vi "Write Attribute.vi"(4 "Private?":bool, 5 "Update Pointer?":bool, 6 "Pointer?":bool, 7 "Linked List ID":string, 8 "error in (no error)":errorcluster, 9 "Attribute":variant, 10 "Attribute Name":string, 11 "Linked List in":refnum<class "Linked List.lvclass">) -> (0 "error out":errorcluster, 1 "Replaced?":bool, 2 "Unique ID":string, 3 "Linked List out":refnum<class "Linked List.lvclass">)   [LabVIEW 2019, in "Linked Lists.lvlib" / "Linked List.lvclass"]
uses:
  <vilib>/gpm_packages/@cs/linked-list/Source/Linked List/Linked List/Linked List.lvclass
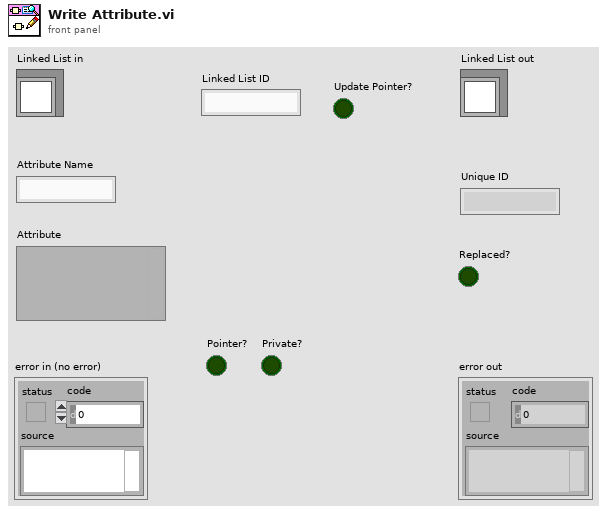
[diagram p1: front panel]
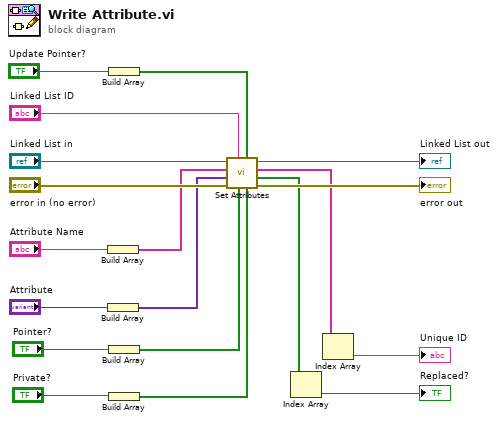
[diagram p0: block diagram]
diagram:
  n1 = Build Array("Attribute Name") -> (w13:string[])
  n2 = Build Array("Attribute") -> (w11:variant[])
  n3 = Build Array("Update Pointer?") -> (w1:bool[])
  n4 = Build Array("Pointer?") -> (w5:bool[])
  n5 = Build Array("Private?") -> (w3:bool[])
  n6 = call <vilib>:"Set Attributes.vi"("Private"=w3, "Update Pointer"=w1, "Pointer"=w5, "Unique ID"="Linked List ID", "error in (no error)"="error in (no error)", "Data"=w11, "Name"=w13, "Linked List in"="Linked List in") -> ("error out"=→"error out":errorcluster, "Replaced?"=w8:bool[], "Unique IDs"=w10:string[], "Linked List out"=→"Linked List out":refnum<class "Linked List.lvclass">)
  n7 = Index Array(array=w8) -> (element=→"Replaced?":bool)  [unwired: 1 in]
  n8 = Index Array(array=w10) -> (element=→"Unique ID":string)  [unwired: 1 in]
